vi "FreqC.Close Message Session.vi"(8 "error in":errorcluster, 11 "FreqC Message Session in":T1) -> (0 "error out":errorcluster)   [LabVIEW 2018]
uses:
  typedefs/FreqC.Message Session.ctl
  typedefs/FreqC.Message.ctl
  typedefs/FreqC.Message Type.ctl
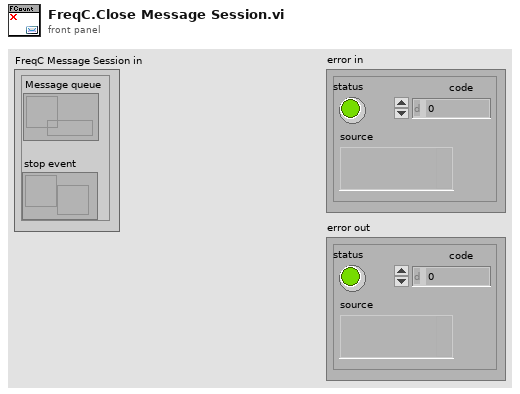
[diagram p1: front panel]
types:
  T1 = typedef "FreqC.Message Session.ctl" = cluster{"Message queue":refnum<queue>, "stop event":refnum<user-event>}
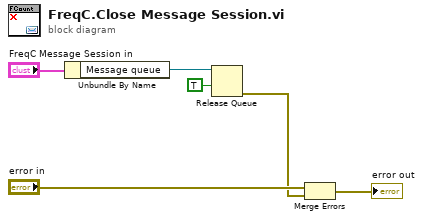
[diagram p0: block diagram]
diagram:
  n1 = Unbundle By Name("FreqC Message Session in") -> ("Message queue"=w5:refnum<queue>)
  n2 = Release Queue(queue=w5, force destroy? (F)=TRUE) -> (error out=w1:errorcluster)  [unwired: 1 in, 2 out]
  n3 = Merge Errors("error in", w1) -> (→"error out":errorcluster)
